vi "RT Main.vi"() -> ()   [LabVIEW 2018]
doc: "The myRIO Custom FPGA Project template acquires button data from the onboard button and displays the button value on a Boolean indicator. The SYS.RDY indicator shows the FPGA status."
uses:
  <vilib>/FPGAPlugInAG/myRIO-1900/niLvFpga_Open_myRIO-1900.vi
  <vilib>/Utility/error.llb/Error Cluster From Error Code.vi
  <vilib>/rvi/errors/niLvFpgaAdjustHostInterfaceError.vi
  <vilib>/FPGAPlugInAG/myRIO-1900/niLvFpga_Run_myRIO-1900.vi
  <vilib>/FPGAPlugInAG/myRIO-1900/niLvFpga_Close_myRIO-1900.vi
  <vilib>/rvi/interface/nirviOpenFPGA/nirviOpenFPGA.xnode
  FPGA Bitfiles/3.0_FPGATarget_FPGA_9hg9oG0pXoA.lvbitx
  FPGA.vi
  <vilib>/rvi/interface/nirviMethod/nirviMethod.xnode
  <vilib>/rvi/interface/nirviReadWriteControl/nirviReadWriteControl.xnode
  <vilib>/rvi/interface/nirviCloseFPGA/nirviCloseFPGA.xnode
  <vilib>/rvi/errors/niLvFpgaMergeErrorWithErrorCode.vi
  <vilib>/FPGAPlugInAG/myRIO-1900/niLvFpga_StartFifo_myRIO-1900.vi
  <vilib>/FPGAPlugInAG/myRIO-1900/niLvFpga_ReadFifo_myRIO-1900.vi
  NiFpgaLv.dll
panel:
  out "Thrust Force":i32[](graph)
  out "torque":i32[](graph)
  out "Timed Out?":bool
  out "error out 2":errorcluster
  in  "stop":bool
  out "error out":errorcluster
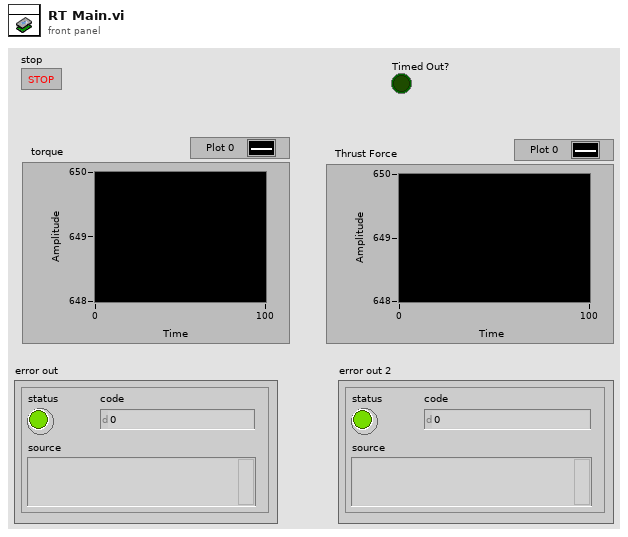
[diagram p1: front panel]
types:
  T1 = enum16{"open", "open or create", "create or replace", "create", "open (read-only)"}
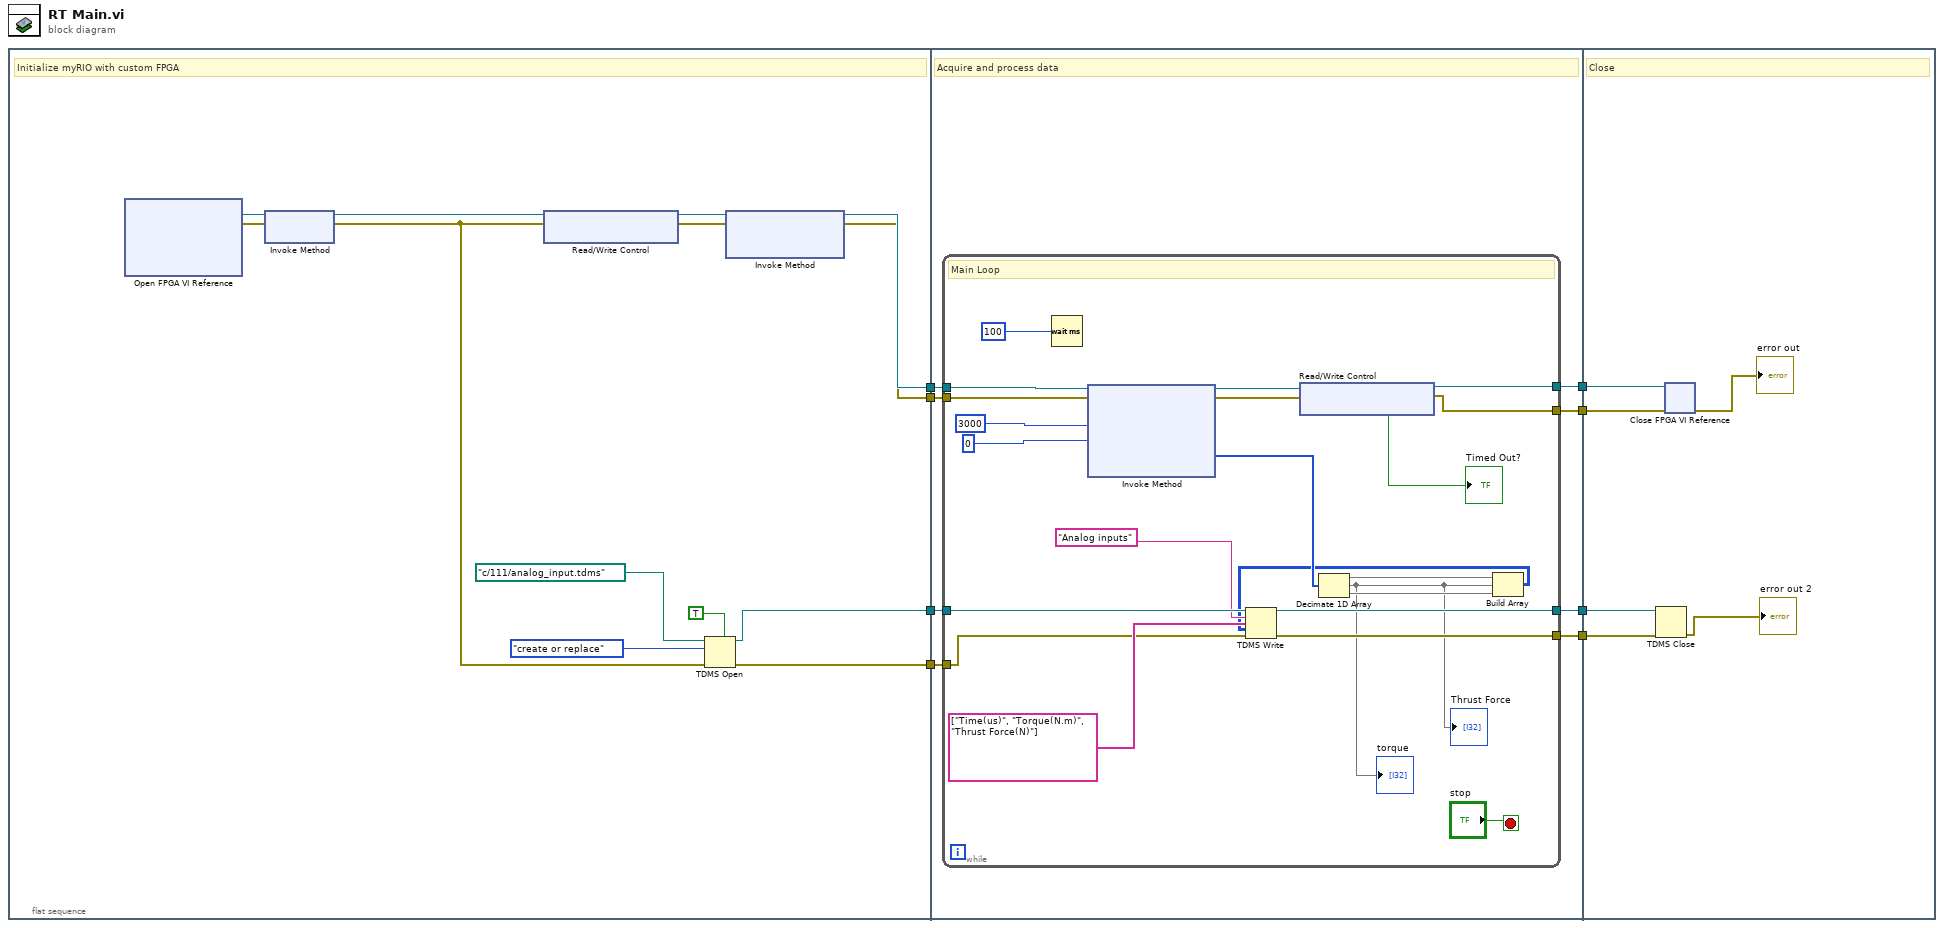
[diagram p0: block diagram]
diagram:
  n1 = flat-sequence {
    tunnel: [w19] -> w8
    tunnel: [w18] -> w7
    tunnel: [w15] -> w4
    tunnel: [w14] -> w3
    tunnel: w8 -> [w29]
    tunnel: w7 -> [w28]
    tunnel: [w27] -> w6
    tunnel: [w26] -> w5
    tunnel: w4 -> [w25]
    tunnel: w3 -> [w24]
    tunnel: [w23] -> w2
    tunnel: [w22] -> w1
    tunnel: w6 -> [w57]
    tunnel: w5 -> [w53]
    tunnel: w2 -> [w56]
    tunnel: w1 -> [w55]
    frame #0 {
      # "Initialize myRIO with custom FPGA"
      n2 = xnode "Open FPGA VI Reference"() -> ("FPGA VI Reference Out"=w21:refnum<k20>, "error out"=w20:errorcluster)  [unwired: 2 in]
      n3 = xnode "Invoke Method"("FPGA VI Reference In"=w21, "error in"=w20) -> ("FPGA VI Reference Out"=w9:refnum<k20>, "error out"=w10:errorcluster)
      n4 = xnode "Read/Write Control"("FPGA VI Reference In"=w9, "error in"=w10) -> ("FPGA VI Reference Out"=w13:refnum<k20>, "error out"=w11:errorcluster)  [unwired: 1 out]
      n5 = TDMS Open(5:TRUE ("create index file? (T)"), 8:w10, 10:T1."create or replace" ("operation (0:open)"), 11:path "c:/111/analog_input.tdms" ("file path")) -> (0:w14:errorcluster, 3:w15:refnum<k34>)  [unwired: 3 in]
      n6 = xnode "Invoke Method"("FPGA VI Reference In"=w13, "error in"=w11) -> ("FPGA VI Reference Out"=w19:refnum<k20>, "error out"=w18:errorcluster)  [unwired: 1 in]
    }
    frame #1 {
      # "Acquire and process data"
      n7 = while {
        tunnel: w29 -> [w51]
        tunnel: w28 -> [w50]
        tunnel: [w45] -> w27
        tunnel: [w44] -> w26
        tunnel: w25 -> [w42]
        tunnel: w24 -> [w36]
        tunnel: [w41] -> w23
        tunnel: [w40] -> w22
        stop <- "stop" stop-if-true
        # "Main Loop"
        n8 = Wait (ms)(milliseconds to wait=u32 100) -> ()  [unwired: 1 out]
        n9 = xnode "Invoke Method"("FPGA VI Reference In"=w51, "error in"=w50, "Number of Elements"=u32 3000, "Timeout (ms)"=0) -> ("FPGA VI Reference Out"=w47:refnum<k20>, "error out"=w46:errorcluster, "Data"=w32:i32[])  [unwired: 1 out]
        n10 = xnode "Read/Write Control"("FPGA VI Reference In"=w47, "error in"=w46) -> ("FPGA VI Reference Out"=w45:refnum<k20>, "error out"=w44:errorcluster, "Timed Out?"=→"Timed Out?":bool)
        n11 = Decimate 1D Array(w32) -> (w34:i32[], w31:i32[], w33:i32[])
        "torque" <- w31
        "Thrust Force" <- w31
        n12 = Build Array(w34, w31, w33) -> (w30:i32[][])
        n13 = TDMS Write(0:w42, 5:"Analog inputs" ("group name in (Untitled)"), 7:string[] ["Time(us)", "Torque(N.m)", "Thrust Force(N)"] ("channel name(s) in (Untitled)"), 9:w30, 11:w36) -> (4:w41:refnum<k34>, 15:w40:errorcluster)  [unwired: 1 in, 2 out]
      }
    }
    frame #2 {
      # "Close"
      n14 = TDMS Close(8:w55, 11:w56) -> (0:→"error out 2":errorcluster)  [unwired: 1 out]
      n15 = xnode "Close FPGA VI Reference"("FPGA VI Reference In"=w57, "error in"=w53) -> ("error out"=→"error out":errorcluster)
    }
  }
